vi "Teleop.vi"(10 "Match Info":T1={"Autonomous Elapsed Seconds"=0.0, "TeleOp Elapsed Seconds"=0.0, "Disabled Elapsed Seconds"=0.0, "Visited Autonomous"=FALSE, "Visited TeleOp"=FALSE, "Visited Disabled"=FALSE, "Autonomous Settings"={"Autonomous Style"=enum."Independent", "VI Refnum"=refnum}}, 11 "Call Context":T2) -> ()   [LabVIEW 2016]
doc: "This VI is called for each TeleOp packet received from the DS where the robot is not disabled. It is often used to read from the joysticks and update I/O or to update setpoints for timed control loops. It should complete and return within 20 milliseconds or it may miss DS packets."
uses:
  <vilib>/Rock Robotics/WPI/DriverStation/WPI_DriverStationDerivedRobotMode.ctl
  <vilib>/Rock Robotics/WPI/DriverStation/WPI_DriverStationMatch Info.ctl
  <vilib>/Rock Robotics/WPI/Solenoid/WPI_SolenoidValue.ctl
  <vilib>/Rock Robotics/WPI/Utilities/WPI_GetSetVariantRefNum.vi
  <vilib>/Rock Robotics/Network Tables/NT Write Boolean Array.vi
  <vilib>/Rock Robotics/Network Tables/NT Write Numeric Array.vi
  <vilib>/Rock Robotics/Network Tables/NT Read Boolean.vi
  <vilib>/Rock Robotics/Network Tables/NT Read Number.vi
  <vilib>/Rock Robotics/WPI/Solenoid/WPI_SolenoidSetEnum.vi
  <vilib>/Rock Robotics/WPI/Solenoid/WPI_SolenoidGetEnum.vi
  <vilib>/Rock Robotics/Network Tables/NT Write Number.vi
panel:
  out "Sample Slider 0":dbl(slide) scale=0.0..5.0
  out "Sample Boolean 1":bool
  out "Sample Boolean 0":bool
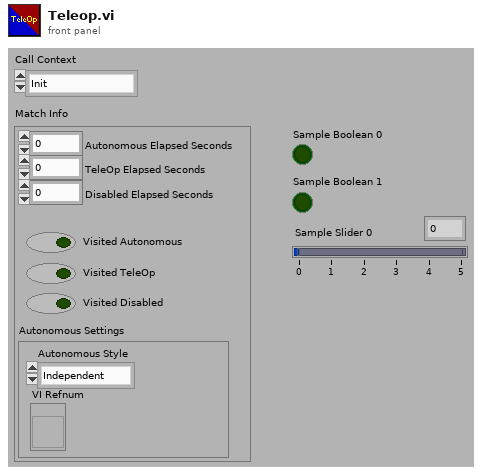
[diagram p1: front panel]
types:
  T1 = typedef "WPI_DriverStationMatch Info.ctl" = cluster{"Autonomous Elapsed Seconds":dbl, "TeleOp Elapsed Seconds":dbl, "Disabled Elapsed Seconds":dbl, "Visited Autonomous":bool, "Visited TeleOp":bool, "Visited Disabled":bool, "Autonomous Settings":cluster{"Autonomous Style":enum16{"Iterative", "Independent"}, "VI Refnum":refnum<vi>}}
  T2 = typedef "WPI_DriverStationDerivedRobotMode.ctl" = enum16{"Init", "Execute", "Stop"}
  T3 = typedef "WPI_SolenoidValue.ctl" = enum16{"Off", "On", "Forward", "Reverse"}
  T4 = typedef "WPI_MotorControlDeviceRef.ctl" = cluster{"DeviceStatus":errorcluster, "Type":T5, "PWM":cluster{"PWM Channel":T6, "DeadBand":T7}, "CAN":cluster{"Device Number":u8, "SetOutput VI Ref":variant, "GetOutput VI Ref":variant, "Enable VI Ref":variant, "Disable VI Ref":variant, "Data":variant}, "Invert":bool}
  T5 = typedef "WPI_MotorControlType.ctl" = enum16{"PWM", "CAN"}
  T6 = typedef "FPGA_DIOPWMChannel.ctl" = enum8{"PWM 0", "PWM 1", "PWM 2", "PWM 3", "PWM 4", "PWM 5", "PWM 6", "PWM 7", "PWM 8", "PWM 9", "PWM MXP 0", "PWM MXP 1", "PWM MXP 2", "PWM MXP 3", "PWM MXP 4", "PWM MXP 5", "PWM MXP 6", "PWM MXP 7", "PWM MXP 8", "PWM MXP 9", "Invalid"}
  T7 = typedef "WPI_PWMDeadband.ctl" = cluster{"Name":string, "maxPositivePwm":i32, "minPositivePwm":i32, "centerPwm":i32, "maxNegativePwm":i32, "minNegativePwm":i32, "angularRange":u16}
  T8 = typedef "WPI_RobotDriveDevRef.ctl" = cluster{"DevStatus":errorcluster, "Motors[]":T4[], "Square Inputs":bool, "Max Output":dbl}
  T9 = typedef "WPI_JoystickDevRef.ctl" = cluster{"Device":T10}
  T10 = typedef "WPI_JoystickDeviceEnum.ctl" = enum16{"USB 0", "USB 1", "USB 2", "USB 3", "USB 4", "USB 5"}
  T11 = typedef "WPI_CANTalonSRX_GlobalStatus.ctl" = cluster{"Applied Throttle":dbl, "Module Enabled":bool, "CAN Error":errorcluster, "Closed Loop Error":dbl, "Forward Limit Switch Closed":bool, "Reverse Limit Switch Closed":bool, "Sensor Position":dbl, "Sensor Velocity":dbl, "Current":dbl, "Sticky Fault - Over Temp":bool, "Sticky Fault - Under Voltage":bool, "Sticky Fault - Forward Limit":bool, "Sticky Fault - Reverse Limit":bool, "Sticky Fault - Forward Soft Limit":bool, "Sticky Fault - Reverse Soft Limit":bool, "Brake is Enabled":bool, "Encoder Position":dbl, "Encoder Velocity":dbl, "Encoder Index Count":dbl, "Encoder A Pin State":bool, "Encoder B Pin State":bool, "Encoder Index Pin State":bool, "Analog In":dbl, "Analog In Velocity":dbl, "Temperature (C)":dbl, "Battery Voltage":dbl, "Control 5 Is Supported":bool, "Current Profile Slot Select":dbl, "Pos Div 8":bool, "Vel Div 4":bool, "Pulse Width Position":i32, "Pulse Width Velocity":i32, "Pulse Width Rise To Rise (us)":i32, "Pulse Width Rise To Fall (us)":i32, "Mot Prof Active Is Under Run":bool, "Mot Prof Active Has Under Run":bool, "Mot Prof Active Is Last":bool, "Mot Prof Active Velocity Only":bool, "Mot Prof Active Is Valid":bool, "Mot Prof Buffer Is Full":bool, "Mot Prof Active Profile Slot Select":i32, "Mot Prof NextID":i32, "Mot Prof Count":i32, "Mot Prof Active Velocity":dbl, "Mot Prof Active Position":dbl, "Mot Prof Output Enable":i32}
  T12 = typedef "WPI_SolenoidDevRef.ctl" = cluster{"DevStatus":errorcluster, "Pneumatics Control Module":u8, "Forward Solenoid Channel":T13, "Reverse Solenoid Channel":T13}
  T13 = typedef "WPI_SolenoidChannel.ctl" = enum8{"Solenoid 0", "Solenoid 1", "Solenoid 2", "Solenoid 3", "Solenoid 4", "Solenoid 5", "Solenoid 6", "Solenoid 7", "Invalid"}
  T14 = typedef "WPI_ServoDeviceRef.ctl" = cluster{"DeviceStatus":errorcluster, "PWM Channel":T6, "DeadBand":T7}
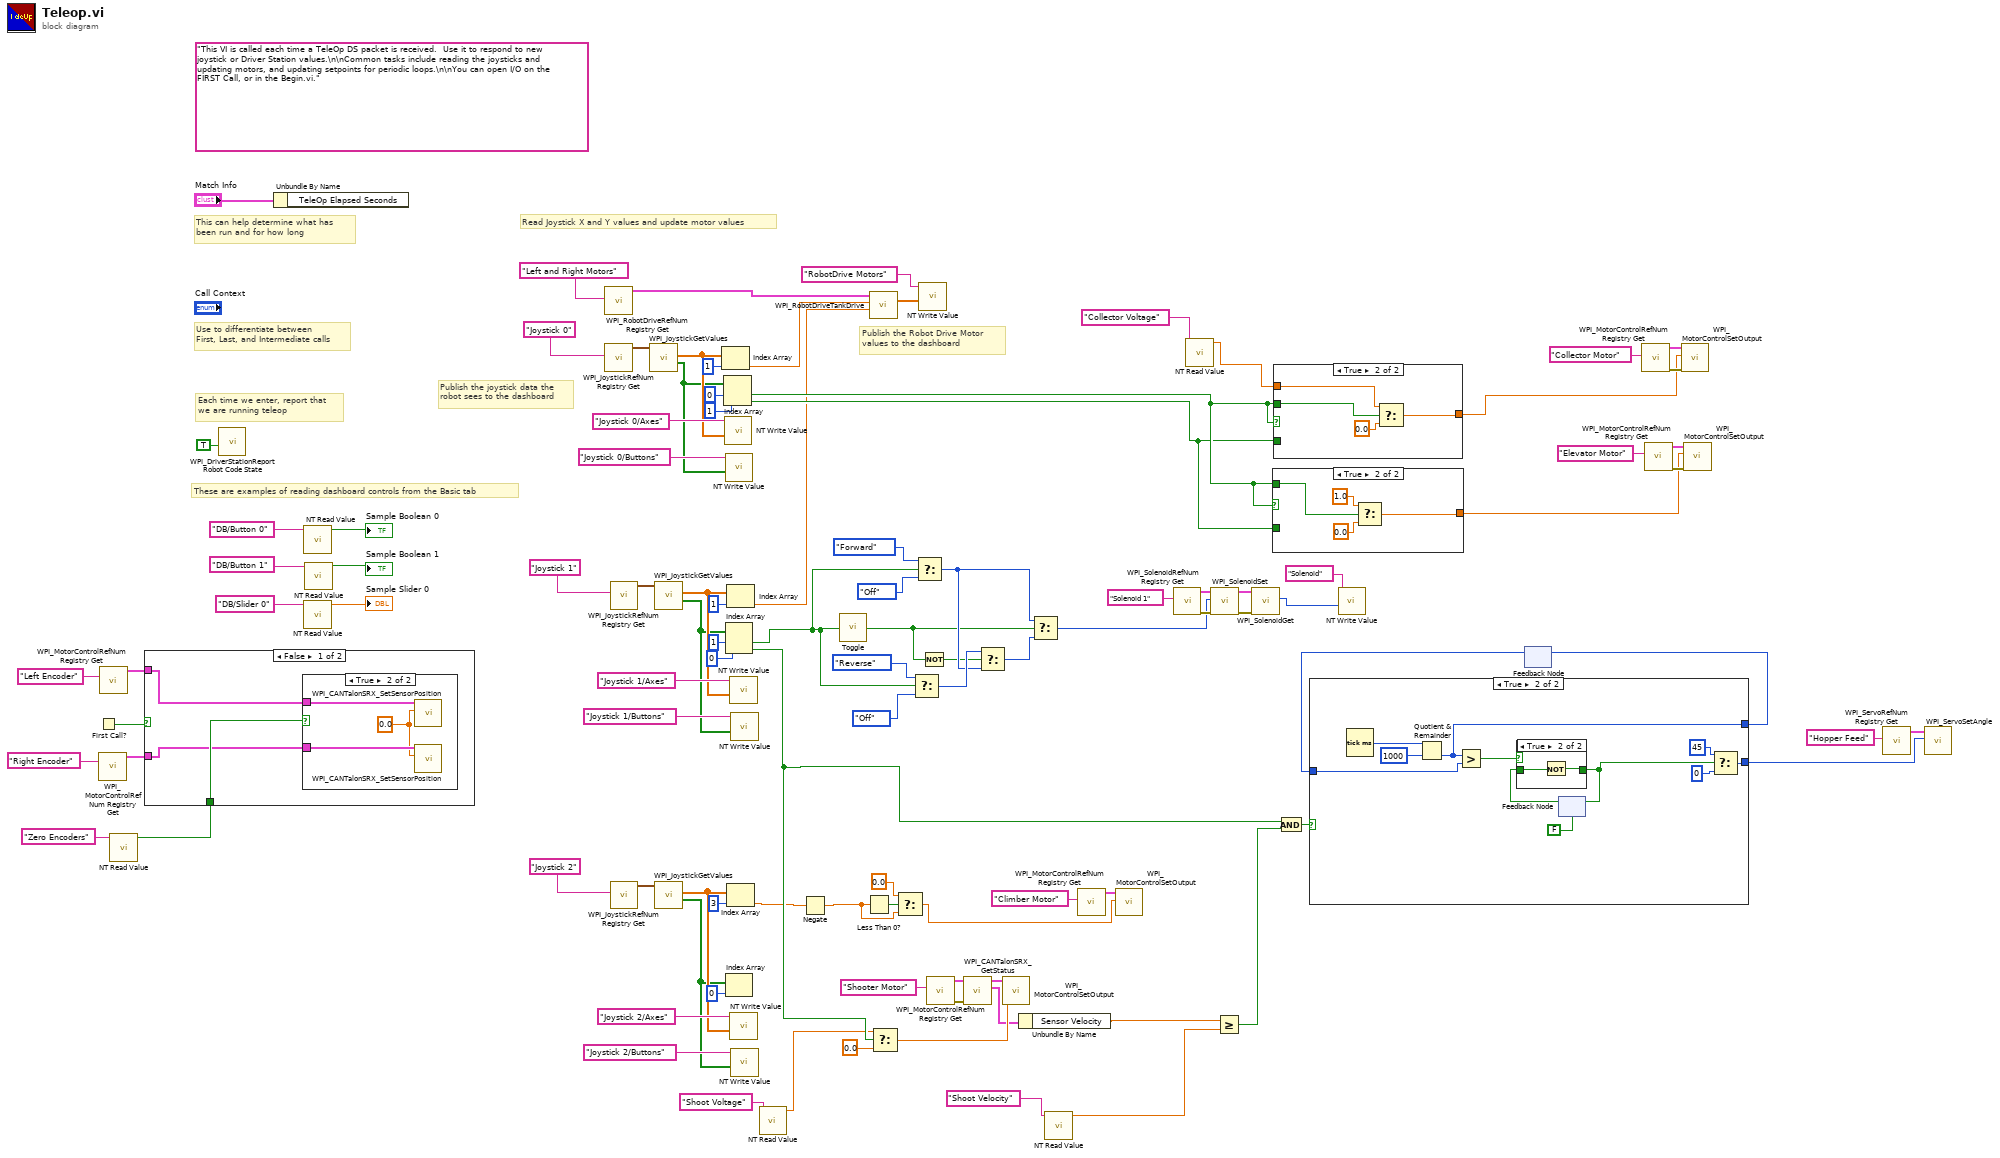
[diagram p0: block diagram]
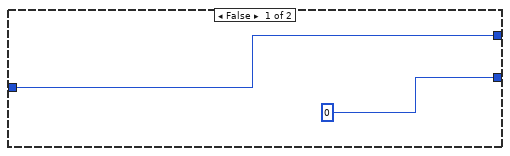
[diagram p2: hidden frame]
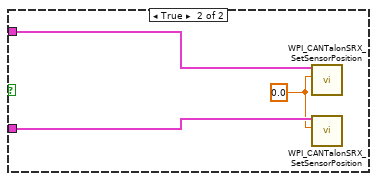
[diagram p5: hidden frame]
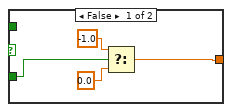
[diagram p6: hidden frame]
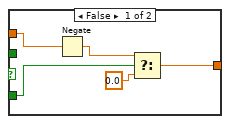
[diagram p7: hidden frame]
diagram:
  (unwired) "This VI is called each time a TeleOp DS packet is received.  Use it to respond to new joystick or Driver Station values.\n\nCommon tasks include reading the joysticks and updating motors, and updating setpoints for periodic loops.\n\nYou can open I/O on the FIRST Call, or in the Begin.vi."
  # "These are examples of reading dashboard controls from the Basic tab"
  # "Publish the Robot Drive Motor\nvalues to the dashboard"
  # "Publish the joystick data the\nrobot sees to the dashboard"
  # "Each time we enter, report that\nwe are running teleop"
  # "Use to differentiate between\nFirst, Last, and Intermediate calls"
  # "This can help determine what has\nbeen run and for how long"
  # "Read Joystick X and Y values and update motor values"
  n1 = First Call?() -> (First Call?: T/F=w27:bool)
  n2 = call <vilib>:"WPI_MotorControlRefNum Registry Get.vi"("refnum name"="Right Encoder") -> ("MotorControlDevRef"=w30:T4)  [unwired: 9 in, 1 out]
  n3 = call <vilib>:"WPI_MotorControlRefNum Registry Get.vi"("refnum name"="Left Encoder") -> ("MotorControlDevRef"=w28:T4)  [unwired: 9 in, 1 out]
  n4 = call-poly <vilib>:"NT Read Value.vi"("Name"="Zero Encoders") -> ("Boolean"=w26:bool)  [unwired: 9 in, 1 out]
  n5 = case shown="False" w27 {
    tunnel: w30 -> [w105 w113]
    tunnel: w28 -> [w106 w112]
    tunnel: w26 -> [w107 _]
    frame False {
      n6 = case shown="True" w107 {
        tunnel: w105 -> [_ w109]
        tunnel: w106 -> [_ w110]
        frame False {
        }
        frame True {
          w108 = 0.0
          n7 = call <vilib>:"WPI_CANTalonSRX_SetSensorPosition.vi"("New Sensor Position"=w108, "CAN Talon SRX Ref"=w110) -> ()  [unwired: 8 in, 2 out]
          n8 = call <vilib>:"WPI_CANTalonSRX_SetSensorPosition.vi"("New Sensor Position"=w108, "CAN Talon SRX Ref"=w109) -> ()  [unwired: 8 in, 2 out]
        }
      }
    }
    frame True {
      w111 = 0.0
      n9 = call <vilib>:"WPI_CANTalonSRX_SetSensorPosition.vi"("New Sensor Position"=w111, "CAN Talon SRX Ref"=w112) -> ()  [unwired: 8 in, 2 out]
      n10 = call <vilib>:"WPI_CANTalonSRX_SetSensorPosition.vi"("New Sensor Position"=w111, "CAN Talon SRX Ref"=w113) -> ()  [unwired: 8 in, 2 out]
    }
  }
  n11 = call <vilib>:"WPI_DriverStationReport Robot Code State.vi"("TeleOp"=TRUE ("Autonomous")) -> ()  [unwired: 10 in, 1 out]
  n12 = Unbundle By Name("Match Info") -> ()  [unwired: 1 out]
  n13 = call-poly <vilib>:"NT Read Value.vi"("Name"="DB/Button 0" ("refnum name")) -> ("Boolean"=→"Sample Boolean 0":bool)  [unwired: 9 in, 1 out]
  n14 = call-poly <vilib>:"NT Read Value.vi"("Name"="DB/Slider 0" ("refnum name")) -> ("Numeric"=→"Sample Slider 0":dbl)  [unwired: 9 in, 1 out]
  n15 = call-poly <vilib>:"NT Read Value.vi"("Name"="DB/Button 1" ("refnum name")) -> ("Boolean"=→"Sample Boolean 1":bool)  [unwired: 9 in, 1 out]
  n16 = call <vilib>:"WPI_RobotDriveRefNum Registry Get.vi"("refnum name"="Left and Right Motors") -> ("RobotDriveDevRef"=w102:T8)  [unwired: 1 in, 9 out]
  n17 = call <vilib>:"WPI_JoystickRefNum Registry Get.vi"("refnum name"="Joystick 0") -> ("JoystickDevRef"=w100:T9)  [unwired: 1 in, 9 out]
  n18 = call <vilib>:"WPI_JoystickRefNum Registry Get.vi"("refnum name"="Joystick 1") -> ("JoystickDevRef"=w87:T9)  [unwired: 1 in, 9 out]
  n19 = call <vilib>:"WPI_JoystickRefNum Registry Get.vi"("refnum name"="Joystick 2") -> ("JoystickDevRef"=w82:T9)  [unwired: 1 in, 9 out]
  n20 = call <vilib>:"WPI_JoystickGetValues.vi"("JoystickDevRef"=w100) -> ("Buttons"=w72:bool[], "Axes"=w96:dbl[])  [unwired: 6 in, 3 out]
  n21 = call <vilib>:"WPI_JoystickGetValues.vi"("JoystickDevRef"=w87) -> ("Buttons"=w52:bool[], "Axes"=w84:dbl[])  [unwired: 6 in, 3 out]
  n22 = call <vilib>:"WPI_JoystickGetValues.vi"("JoystickDevRef"=w82) -> ("Buttons"=w48:bool[], "Axes"=w79:dbl[])  [unwired: 6 in, 3 out]
  n23 = Index Array(array=w96, index=1) -> (element=w34:dbl)
  n24 = Index Array(array=w72, index #1=0 ("index"), index #2=1 ("index")) -> (element #1=w40:bool, element #2=w39:bool)
  n25 = call-poly <vilib>:"NT Write Value.vi"("Numeric Array"=w96, "Name"="Joystick 0/Axes") -> ()  [unwired: 9 in, 1 out]
  n26 = call-poly <vilib>:"NT Write Value.vi"("Boolean Array"=w72, "Name"="Joystick 0/Buttons") -> ()  [unwired: 9 in, 1 out]
  n27 = Index Array(array=w52, index #1=1 ("index"), index #2=0 ("index")) -> (element #1=w53:bool, element #2=w14:bool)
  n28 = Index Array(array=w48, index=0) -> ()  [unwired: 1 out]
  n29 = Index Array(array=w84, index=1) -> (element=w35:dbl)
  n30 = Index Array(array=w79, index=3) -> (element=w6:dbl)
  n31 = call-poly <vilib>:"NT Write Value.vi"("Numeric Array"=w84, "Name"="Joystick 1/Axes") -> ()  [unwired: 9 in, 1 out]
  n32 = call-poly <vilib>:"NT Write Value.vi"("Numeric Array"=w79, "Name"="Joystick 2/Axes") -> ()  [unwired: 9 in, 1 out]
  n33 = call-poly <vilib>:"NT Write Value.vi"("Boolean Array"=w52, "Name"="Joystick 1/Buttons") -> ()  [unwired: 9 in, 1 out]
  n34 = call-poly <vilib>:"NT Write Value.vi"("Boolean Array"=w48, "Name"="Joystick 2/Buttons") -> ()  [unwired: 9 in, 1 out]
  n35 = call-poly <vilib>:"NT Read Value.vi"("Name"="Shoot Voltage") -> ("Numeric"=w1:dbl)  [unwired: 9 in, 1 out]
  n36 = Negate(x=w6) -> (-x=w5:dbl)
  n37 = call "Toggle.vi"("Input"=w53) -> ("Output"=w55:bool)
  n38 = Less Than 0?(x=w5) -> (x < 0?=w38:bool)
  n39 = call <vilib>:"WPI_RobotDriveTankDrive.vi"("Right axis value"=w35, "Left axis value"=w34, "RobotDriveDevRef"=w102) -> ("Motor Values"=w89:dbl[])  [unwired: 6 in, 2 out]
  n40 = Select(t=w1, s=w14, f=0.0) -> (s? t:f=w21:dbl)
  n41 = Select(t=0.0 ("f"), s=w38, f=w5) -> (s? t:f=w37:dbl)
  n42 = Select(t=WPI_SolenoidValue."Reverse" ("Value"), s=w53, f=WPI_SolenoidValue."Off") -> (s? t:f=w58:T3)
  n43 = Select(t=WPI_SolenoidValue."Forward" ("Value"), s=w53, f=WPI_SolenoidValue."Off" ("Value")) -> (s? t:f=w56:T3)
  n44 = call-poly <vilib>:"NT Write Value.vi"("Numeric Array"=w89, "Name"="RobotDrive Motors") -> ()  [unwired: 9 in, 1 out]
  n45 = Not(x=w55) -> (.not. x?=w54:bool)
  n46 = call <vilib>:"WPI_MotorControlRefNum Registry Get.vi"("refnum name"="Shooter Motor") -> ("error out"=w25:errorcluster, "MotorControlDevRef"=w24:T4)  [unwired: 9 in]
  n47 = call <vilib>:"WPI_CANTalonSRX_GetStatus.vi"("error in (no error)"=w25, "CAN Talon SRX Ref"=w24) -> ("Talon SRX Status"=w20:T11, "CAN Talon SRX Ref"=w23:T4)  [unwired: 7 in, 1 out]
  n48 = Select(t=w58, s=w54, f=w56) -> (s? t:f=w57:T3)
  n49 = call <vilib>:"WPI_MotorControlSetOutput.vi"("Output"=w21, "MotorControlDevRef"=w23) -> ()  [unwired: 7 in, 3 out]
  n50 = Unbundle By Name(w20) -> ("Sensor Velocity"=w12:dbl)
  n51 = Select(t=w56, s=w55, f=w57) -> (s? t:f=w60:T3)
  n52 = call-poly <vilib>:"NT Read Value.vi"("Name"="Shoot Velocity") -> ("Numeric"=w2:dbl)  [unwired: 9 in, 1 out]
  n53 = call <vilib>:"WPI_MotorControlRefNum Registry Get.vi"("refnum name"="Climber Motor") -> ("MotorControlDevRef"=w74:T4)  [unwired: 9 in, 1 out]
  n54 = call <vilib>:"WPI_MotorControlSetOutput.vi"("Output"=w37, "MotorControlDevRef"=w74) -> ()  [unwired: 7 in, 3 out]
  n55 = call <vilib>:"WPI_SolenoidRefNum Registry Get.vi"("refnum name"="Solenoid 1") -> ("error out"=w65:errorcluster, "SolenoidDevRef"=w64:T12)  [unwired: 9 in]
  n56 = call-poly <vilib>:"NT Read Value.vi"("Name"="Collector Voltage") -> ("Numeric"=w49:dbl)  [unwired: 9 in, 1 out]
  n57 = call-poly <vilib>:"WPI_SolenoidSet.vi"("error in (no error)"=w65, "Value"=w60, "SolenoidDevRef"=w64) -> ("error out"=w10:errorcluster, "SolenoidDevRef"=w9:T12)  [unwired: 7 in]
  n58 = Greater Or Equal?(x=w12, y=w2) -> (x >= y?=w13:bool)
  n59 = call-poly <vilib>:"WPI_SolenoidGet.vi"("error in (no error)"=w10, "SolenoidDevRef"=w9) -> ("Value"=w8:T3)  [unwired: 7 in, 2 out]
  n60 = case shown="True" w40 {
    tunnel: [w114 w121] -> w41
    tunnel: w40 -> [_ w118]
    tunnel: w39 -> [w117 _]
    frame False {
      n61 = Select(t=-1.0, s=w117, f=0.0) -> (s? t:f=w114:dbl)
    }
    frame True {
      n62 = Select(t=1.0, s=w118, f=0.0) -> (s? t:f=w121:dbl)
    }
  }
  n63 = case shown="True" w40 {
    tunnel: w40 -> [_ w130]
    tunnel: w39 -> [w125 _]
    tunnel: w49 -> [w124 w128]
    tunnel: [w122 w127] -> w42
    frame False {
      n64 = Negate(x=w124) -> (-x=w123:dbl)
      n65 = Select(t=w123, s=w125, f=0.0) -> (s? t:f=w122:dbl)
    }
    frame True {
      n66 = Select(t=w128, s=w130, f=0.0) -> (s? t:f=w127:dbl)
    }
  }
  n67 = And(x=w14, y=w13) -> (x .and. y?=w17:bool)
  n68 = call-poly <vilib>:"NT Write Value.vi"("Numeric"=w8, "Name"="Solenoid") -> ()  [unwired: 9 in, 1 out]
  n69 = feedback #1() -> (w18:u32)  [unwired: 1 in]
  n70 = case shown="True" w17 {
    tunnel: [0 ("Angle") w143] -> w11
    tunnel: w18 -> [w131 w134]
    tunnel: [w131 w133] -> w19
    frame False {
    }
    frame True {
      n71 = Tick Count (ms)() -> (millisecond timer value=w140:u32)
      n72 = Quotient & Remainder(x=w140, y=u32 1000) -> (floor(x/y)=w133:u32)  [unwired: 1 out]
      n73 = Greater?(x=w133, y=w134) -> (0:w135:bool)
      n74 = feedback #2(FALSE) -> (w137:bool)
      n75 = case shown="True" w135 {
        tunnel: w137 -> [w144 w146]
        tunnel: [w144 w145] -> w138
        frame False {
        }
        frame True {
          n76 = Not(x=w146) -> (.not. x?=w145:bool)
        }
      }
      n77 = feedback-in #2(w138) -> ()
      n78 = Select(t=45 ("Angle"), s=w138, f=0 ("Angle")) -> (s? t:f=w143:i32)
    }
  }
  n79 = feedback-in #1(w19) -> ()
  n80 = call <vilib>:"WPI_MotorControlRefNum Registry Get.vi"("refnum name"="Collector Motor") -> ("error out"=w69:errorcluster, "MotorControlDevRef"=w67:T4)  [unwired: 9 in]
  n81 = call <vilib>:"WPI_MotorControlRefNum Registry Get.vi"("refnum name"="Elevator Motor") -> ("error out"=w45:errorcluster, "MotorControlDevRef"=w43:T4)  [unwired: 9 in]
  n82 = call <vilib>:"WPI_MotorControlSetOutput.vi"("error in (no error)"=w69, "Output"=w42, "MotorControlDevRef"=w67) -> ()  [unwired: 6 in, 3 out]
  n83 = call <vilib>:"WPI_MotorControlSetOutput.vi"("error in (no error)"=w45, "Output"=w41, "MotorControlDevRef"=w43) -> ()  [unwired: 6 in, 3 out]
  n84 = call <vilib>:"WPI_ServoRefNum Registry Get.vi"("refnum name"="Hopper Feed") -> ("ServoDeviceRef"=w15:T14)  [unwired: 9 in, 1 out]
  n85 = call <vilib>:"WPI_ServoSetAngle.vi"("Angle"=w11, "ServoDeviceRef"=w15) -> ()  [unwired: 8 in, 2 out]
